vi "TIO Stream Write_Ser.vi"(7 "error in (no error)":errorcluster, 8 "Type":T1(ring)=enum."RPC Request", 9 "Payload":string, 10 "Nom de ressource VISA":refnum<visa-resource-name>) -> (0 "error out":errorcluster, 3 "Nom de ressource VISA Out":refnum<visa-resource-name>)   [LabVIEW 2010]
uses:
  <userlib>/TIO Library 2010/TIO SLIP Encode.vi
  <userlib>/TIO Library 2010/TIO Serial Checksum CRC32.vi
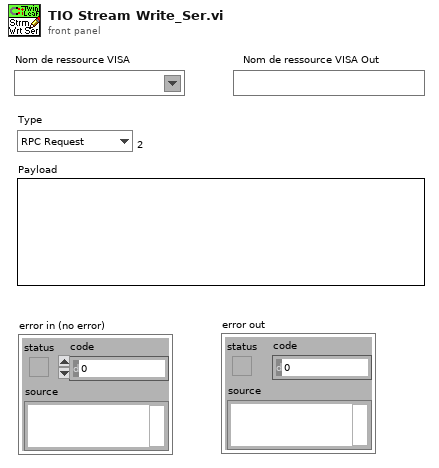
[diagram p1: front panel]
types:
  T1 = enum8{"Invalid", "Log", "RPC Request", "RPC Reply", "RPC Error", "Stream Description", "User"}
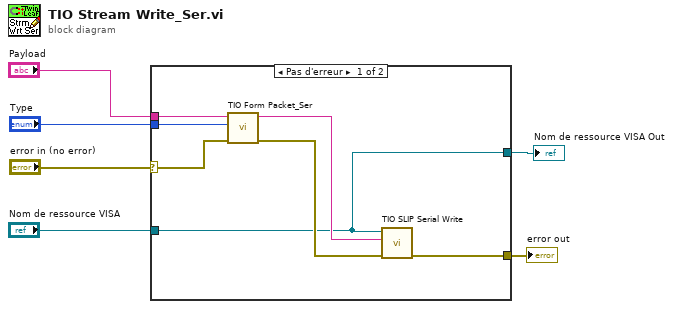
[diagram p0: block diagram]
diagram:
  n1 = case shown="Pas d'erreur" "error in (no error)" {
    selector: "error in (no error)" -> [w8 w15]
    tunnel: [w13 w15] -> w6
    tunnel: "Payload" -> [w12 _]
    tunnel: "Type" -> [w10 _]
    tunnel: "Nom de ressource VISA" -> [w7 w14]
    tunnel: [w7 w14] -> w1
    frame No Error {
      n2 = call <userlib>:"TIO Form Packet_Ser.vi"("error in (no error)"=w8, "Type"=w10, "Payload"=w12) -> ("error out"=w9:errorcluster, "Packet out"=w11:string)  [unwired: 7 in]
      n3 = call <userlib>:"TIO SLIP Serial Write.vi"("error in (no error)"=w9, "Data"=w11, "VISA Refnum in"=w7) -> ("error out"=w13:errorcluster)  [unwired: 8 in]
    }
    frame Error {
    }
  }
  "error out" <- w6
  "Nom de ressource VISA Out" <- w1
